vi "LS370_Queue_Commands.vi"(1 "Control":T1, 2 "Last Status":T1, 3 "Queue":refnum<queue>) -> (0 "New Status":T1)   [LabVIEW 2016]
uses:
  LS370/LS370-Control.ctl
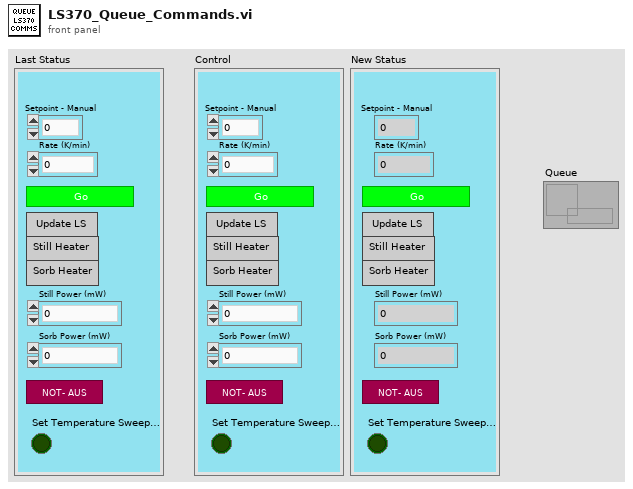
[diagram p1: front panel]
types:
  T1 = typedef "LS370-Control.ctl" = cluster{"Disable Heater":bool, "Activate Tsweep":bool, "Update Lakeshores":bool, "Setpoint - Manual":dbl, "Rate (K/min)":dbl, "Sorb Power (mW)":dbl, "Still Power (mW)":dbl, "Sorb Heater":bool, "Still Heater":bool, "Set Temperature Sweep Main":bool}
  T2 = cluster{"Disable Heater":bool, "Activate Tsweep":bool, "Update Lakeshores":bool, "Setpoint - Manual":bool, "Rate (K/min)":bool, "Sorb Power (mW)":bool, "Still Power (mW)":bool, "Sorb Heater":bool, "Still Heater":bool, "Set Temperature Sweep Main":bool}
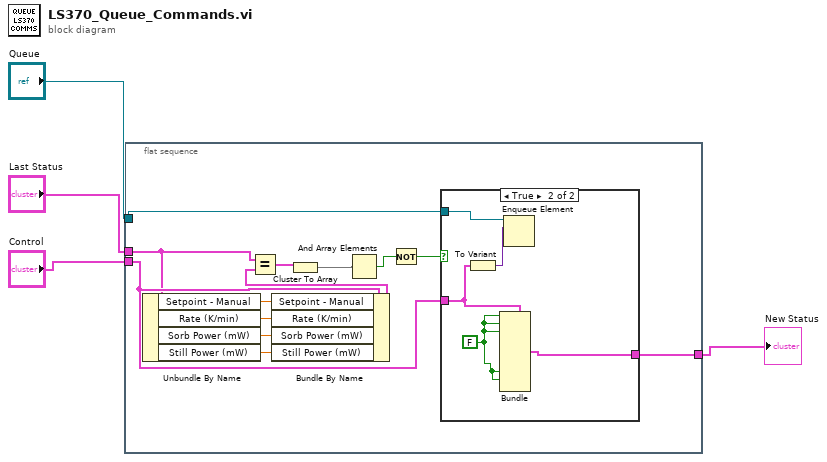
[diagram p0: block diagram]
diagram:
  n1 = flat-sequence {
    tunnel: "Queue" -> [w17]
    tunnel: "Control" -> [w11]
    tunnel: "Last Status" -> [w9]
    tunnel: [w12] -> w1
    frame #0 {
      n2 = Unbundle By Name(w9) -> ("Setpoint - Manual"=w8:dbl, "Rate (K/min)"=w7:dbl, "Sorb Power (mW)"=w6:dbl, "Still Power (mW)"=w5:dbl)
      n3 = Bundle By Name(cluster=w11, "Setpoint - Manual"=w8, "Rate (K/min)"=w7, "Sorb Power (mW)"=w6, "Still Power (mW)"=w5) -> (w10:T1)
      n4 = Equal?(x=w9, y=w10) -> (x = y?=w13:T2)
      n5 = Cluster To Array(cluster=w13) -> (array=w16:bool[])
      n6 = And Array Elements(Boolean array=w16) -> (logical AND=w15:bool)
      n7 = Not(x=w15) -> (.not. x?=w14:bool)
      n8 = case shown="True" w14 {
        tunnel: w17 -> [_ w23]
        tunnel: w11 -> [w18 w21]
        tunnel: [w18 w20] -> w12
        frame False {
        }
        frame True {
          w19 = FALSE
          n9 = To Variant(anything=w21) -> (Variant=w22:variant)
          n10 = Bundle(cluster=w21, "Disable Heater"=w19, "Activate Tsweep"=w19, "Update Lakeshores"=w19, "Sorb Heater"=w19, "Still Heater"=w19) -> (w20:T1)  [unwired: 5 in]
          n11 = Enqueue Element(queue=w23, element=w22) -> ()  [unwired: 2 in, 3 out]
        }
      }
    }
  }
  "New Status" <- w1
